vi "currentExperimentSettings.vi"(8 "error in (no error)":errorcluster, 11 "small?":bool) -> (0 "error out":errorcluster, 1 "Last Name":string, 2 "Last Description":string, 3 "output cluster":T1, 4 "Experiment ID":u64, 5 "Group ID":u64)   [LabVIEW 2013]
doc: "Displays a standard dialog box that prompts users to enter information, such as a user name and password.\n--------------------\n\nThis Express VI is configured as follows:\n\nMessage to Display to the User:Please Enter Experiment Settings Information For Database Storage.\nThe inputs are: \nNumber: Please Enter Group ID\nText Entry Box: Please Enter Tags:\nText Entry Box: Please Enter Experiment Description:"
uses:
  Public API/DisplayExperimentSetting.ctl
  <vilib>/addons/database/_DB Variant To Data/Database Variant To Data.xnode
panel:
  # "Experiment Status:"
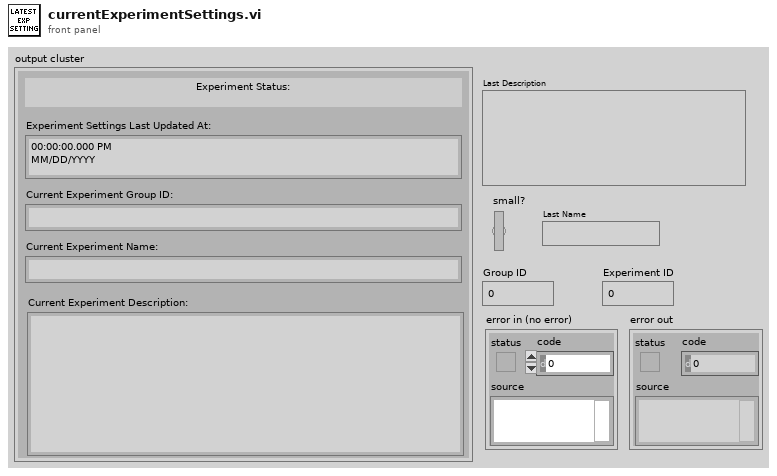
[diagram p1: front panel]
types:
  T1 = typedef "DisplayExperimentSetting.ctl" = cluster{"Current Experiment Name:":string, "Current Experiment Description:":string, "Current Experiment Group ID:":string, "Experiment Settings Last Updated At:":timestamp}
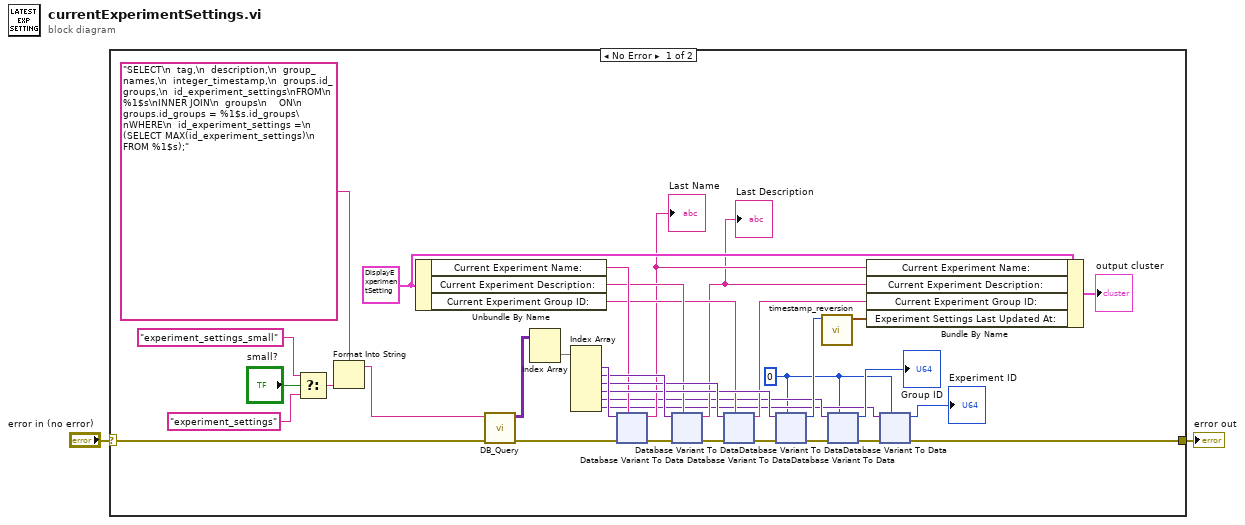
[diagram p0: block diagram]
diagram:
  n1 = case shown="No Error" "error in (no error)" {
    selector: "error in (no error)" -> [w7 w230]
    tunnel: [w4 w230] -> w1
    frame No Error {
      w12 = u64 0 ("Experiment settings ID")
      w26 = T1 {"Current Experiment Name:"="", "Current Experiment Description:"="", "Current Experiment Group ID:"="", "Experiment Settings Last Updated At:"=timestamp(0 s since 1904-01-01)} ("Experiment Settings")
      n2 = Select(t="experiment_settings_small", s="small?", f="experiment_settings") -> (s? t:f=w10:string)
      n3 = Format Into String(format string="SELECT\n  tag,\n  description,\n  group_names,\n  integer_timestamp,\n  groups.id_groups,\n  id_experiment_settings\nFROM\n  %1$s\nINNER JOIN\n  groups\n    ON\n  groups.id_groups = %1$s.id_groups\nWHERE\n  id_experiment_settings =\n   (SELECT MAX(id_experiment_settings)\n    FROM %1$s);" ("SQL query"), w10) -> (resulting string=w3:string)  [unwired: 2 in, 1 out]
      n4 = Unbundle By Name(w26) -> ("Current Experiment Name:"=w25:string, "Current Experiment Description:"=w23:string, "Current Experiment Group ID:"=w22:string)
      n5 = call "DB_Query.vi"("error in (no error)"=w7, "Parameterized Query"=w3) -> ("error out"=w6:errorcluster, "Results"=w5:variant[][])  [unwired: 7 in, 1 out]
      n6 = Index Array(array=w5) -> (element=w27:variant[])  [unwired: 2 in]
      n7 = Index Array(array=w27) -> (element #1=w34:variant, element #2=w33:variant, element #3=w29:variant, element #4=w28:variant, element #5=w14:variant, element #6=w13:variant)  [unwired: 6 in]
      n8 = xnode "Database Variant To Data"("database variant"=w34, "error in (no error)"=w6, "type"=w25) -> ("data"=w20:string, "error out"=w32:errorcluster)
      "Last Name" <- w20
      n9 = xnode "Database Variant To Data"("database variant"=w33, "error in (no error)"=w32, "type"=w23) -> ("data"=w19:string, "error out"=w31:errorcluster)
      "Last Description" <- w19
      n10 = xnode "Database Variant To Data"("database variant"=w29, "error in (no error)"=w31, "type"=w22) -> ("data"=w21:string, "error out"=w30:errorcluster)
      n11 = xnode "Database Variant To Data"("database variant"=w28, "error in (no error)"=w30, "type"=w12) -> ("data"=w24:u64, "error out"=w18:errorcluster)
      n12 = call "timestamp_reversion.vi"("Integer Timestamp"=w24) -> ("time stamp"=w37:timestamp)  [unwired: 8 in, 1 out]
      n13 = xnode "Database Variant To Data"("database variant"=w14, "error in (no error)"=w18, "type"=w12) -> ("data"=→"Group ID":u64, "error out"=w17:errorcluster)
      n14 = Bundle By Name(cluster=w26, "Current Experiment Name:"=w20, "Current Experiment Description:"=w19, "Current Experiment Group ID:"=w21, "Experiment Settings Last Updated At:"=w37) -> (→"output cluster":T1)
      n15 = xnode "Database Variant To Data"("database variant"=w13, "error in (no error)"=w17, "type"=w12) -> ("data"=→"Experiment ID":u64, "error out"=w4:errorcluster)
    }
    frame Error {
    }
  }
  "error out" <- w1
